vi "WriteRead SPI.vi"(4 "CS Active Low (T)":bool=TRUE, 5 "CS Pin (None)":i32=-1, 7 "Bus":u8, 8 "error in (no error)":errorcluster, 10 "Write":string, 11 "VISA resource name in":refnum<visa-resource-name>) -> (0 "error out":errorcluster, 1 "Read":string, 3 "VISA resource name":refnum<visa-resource-name>)   [LabVIEW 2023, in "CTI-Visa.lvlib"]
uses:
  CTI-Visa.lvlib
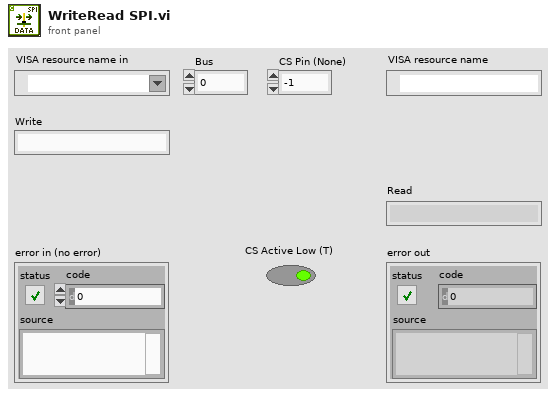
[diagram p1: front panel]
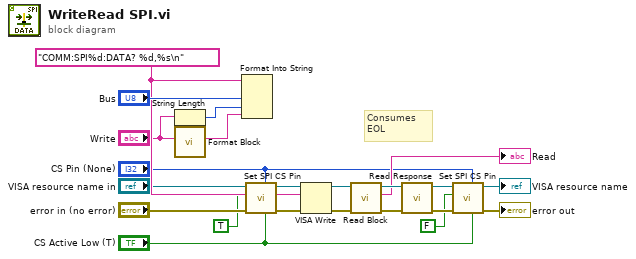
[diagram p0: block diagram]
diagram:
  w19 = "COMM:SPI%d:DATA? %d,%s\n" ("format string")
  # "Consumes EOL"
  n1 = String Length(string="Write") -> (length=w12:i32)
  n2 = call "Format Block.vi"("Data Block"="Write") -> ("Formatted Block"=w11:string)  [unwired: 10 in]
  n3 = Format Into String(format string=w19, "Bus", w12, w11) -> ()  [unwired: 2 in, 2 out]
  n4 = call "Set SPI CS Pin.vi"("CS Active Low (T)"="CS Active Low (T)", "CS GPIO"="CS Pin (None)", "error in (no error)"="error in (no error)", "CS Active"=TRUE, "VISA resource name in"="VISA resource name in") -> ("error out"=w8:errorcluster, "VISA resource name"=w7:refnum<visa-resource-name>)  [unwired: 5 in]
  n5 = VISA Write(VISA resource name=w7, write buffer=w19, error in (no error)=w8) -> (VISA resource name out=w17:refnum<visa-resource-name>, error out=w18:errorcluster)  [unwired: 1 out]
  n6 = call "Read Block.vi"("error in (no error)"=w18, "VISA resource name in"=w17) -> ("error out"=w16:errorcluster, "Data"=→"Read":string, "VISA resource name"=w15:refnum<visa-resource-name>)  [unwired: 7 in]
  n7 = call "Read Response.vi"("error in (no error)"=w16, "VISA resource name in"=w15) -> ("error out"=w21:errorcluster, "VISA resource name"=w5:refnum<visa-resource-name>)  [unwired: 7 in, 1 out]
  n8 = call "Set SPI CS Pin.vi"("CS Active Low (T)"="CS Active Low (T)", "CS GPIO"="CS Pin (None)", "error in (no error)"=w21, "CS Active"=FALSE, "VISA resource name in"=w5) -> ("error out"=→"error out":errorcluster, "VISA resource name"=→"VISA resource name":refnum<visa-resource-name>)  [unwired: 5 in]
